vi "SP Get Frequency Components from Waveform.vi"(0 "Waveform":waveform(dbl)={"t0"=timestamp(0 s since 1904-01-01), "dt"=0.0, "Y"=[]}) -> (1 "F0":dbl, 2 "dF":dbl, 3 "N":i32)   [LabVIEW 2011]
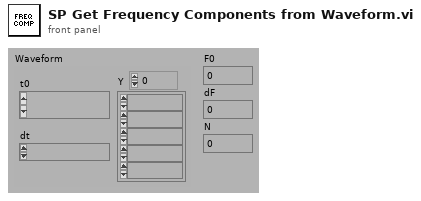
[diagram p1: front panel]
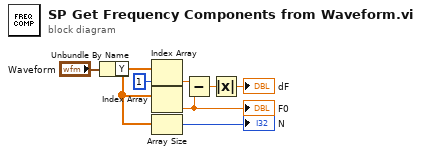
[diagram p0: block diagram]
diagram:
  n1 = Unbundle By Name("Waveform") -> ("Y"=w2:dbl[])
  n2 = Index Array(array=w2, index=1) -> (element=w6:dbl)
  n3 = Index Array(array=w2) -> (element=w5:dbl)  [unwired: 1 in]
  "F0" <- w5
  n4 = Array Size(array=w2) -> (size(s)=→"N":i32)
  n5 = Subtract(x=w6, y=w5) -> (x-y=w4:dbl)
  n6 = Absolute Value(x=w4) -> (abs(x)=→"dF":dbl)
